vi "ti2_setYPos.vi"(8 "error in (no error)":errorcluster, 10 "speed":i32=4, 11 "y Position (um)":dbl) -> (0 "error out":errorcluster)   [LabVIEW 2022 SP3, in "ti2lv.lvlib"]
uses:
  ti2lv.lvlib
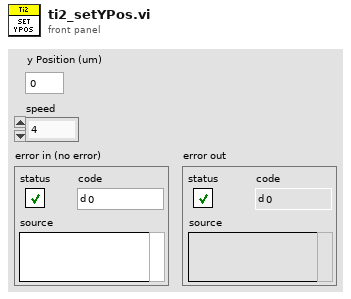
[diagram p1: front panel]
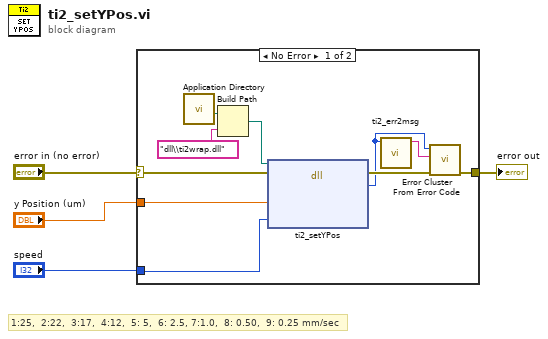
[diagram p0: block diagram]
diagram:
  # "1:25,  2:22, \t3:17,  4:12,\t\t5: 5,  6: 2.5,\t7:1.0,  8: 0.50,  9: 0.25 mm/sec"
  n1 = case shown="No Error" "error in (no error)" {
    selector: "error in (no error)" -> [w13 w15]
    tunnel: [w14 w15] -> w4
    tunnel: "y Position (um)" -> [w9 _]
    tunnel: "speed" -> [w8 _]
    frame No Error {
      n2 = call <vilib>:"Application Directory.vi"() -> ("Application Directory"=w6:path)
      n3 = Build Path(base path=w6, name or relative path="dll\\ti2wrap.dll") -> (appended path=w5:path)
      n4 = dll-call lib="?" fn="ti2_setYPos"(path in=w5, error in=w13, "yPos_um"=w9, "speed"=w8) -> (error out=w12:errorcluster, "return type"=w11:i32)  [unwired: 3 in, 1 out]
      n5 = call "ti2_err2msg.vi"("Error Code"=w11) -> ("Error Message"=w10:string)  [unwired: 10 in]
      n6 = call <vilib>:"Error Cluster From Error Code.vi"("error in (no error)"=w12, "error message (\"\")"=w10, "error code (0)"=w11) -> ("error out"=w14:errorcluster)  [unwired: 6 in]
    }
    frame Error {
    }
  }
  "error out" <- w4
